vi "Main2.vi"() -> ()   [LabVIEW 2020]
uses:
  SuportVI2/Message Queue/Message Queue.lvlib
  SuportVI2/User Event - Stop/User Event - Stop.lvlib
  <vilib>/ErrorRing/Error Ring.xnode
  <vilib>/Utility/error.llb/Error Cluster From Error Code.vi
  <vilib>/userdefined/High Color/IMAQdx.ctl
  <vilib>/vision/Image Controls.llb/IMAQ Image.ctl
  <vilib>/vision/driver/NI_Vision_Acquisition_Software.lvlib
  Add/DAQ AO Sinus Config.ctl
  <vilib>/DAQmx/write.llb/DAQmx Write (Analog Wfm 1Chan NSamp).vi
  Desktop/QMH/ContAcqQMH_Lab/controls/Daqtypedef.ctl
  <vilib>/DAQmx/read.llb/DAQmx Read (Analog Wfm 1Chan NSamp).vi
panel:
  out "Waveform Graph":waveform(dbl)(graph)
  out "DB Data":T1
  out "Status Line 2":string
  in  "Generator Configuration":T2
  out "Image":T3(plugin-control)
  in  "Camera Config":cluster{"Camera Select":T4}
  in  "Exit":bool
  in  "Stop Camera":bool
  in  "Start Camera":bool
  out "Status Line":string
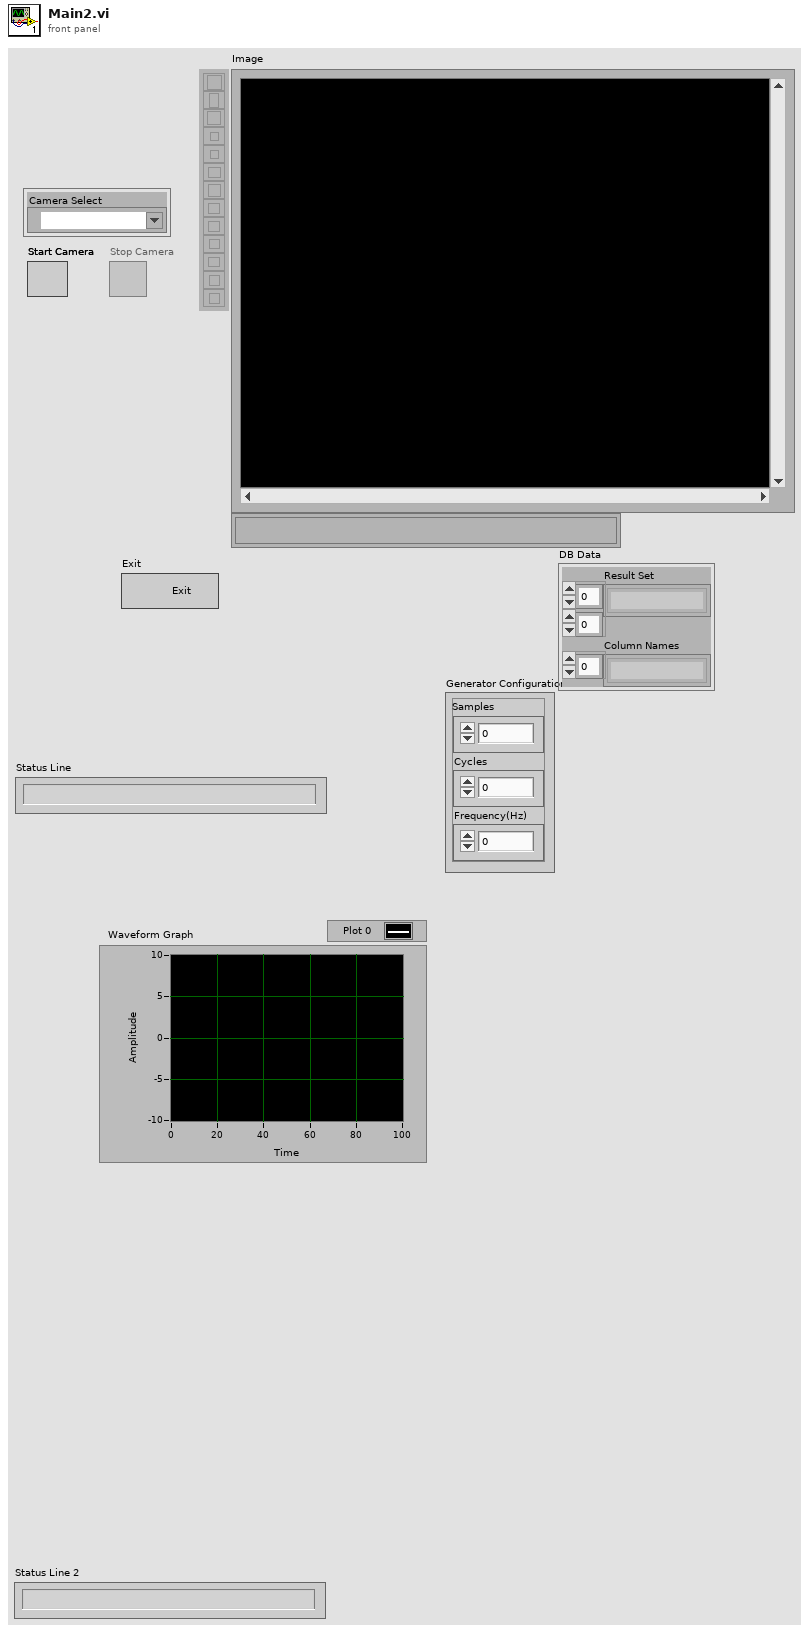
[diagram p1: front panel]
types:
  T1 = cluster{"Result Set":string[][], "Column Names":string[]}
  T2 = typedef "DAQ AO Sinus Config.ctl" = cluster{"Samples":i32, "Cycles":i32, "Frequency(Hz)":dbl}
  T3 = typedef "IMAQ Image.ctl" = refnum<image>
  T4 = typedef "IMAQdx.ctl" = refnum<k21>
  T5 = cluster{"DAQmx Channel":T2, "DAQmx Task":refnum<k21>, "DB Data":cluster{"Result Set":string[][], "Column Names":string[]}}
  T6 = typedef "Daqtypedef.ctl" = cluster{"PhysicalChanName":tag, "AI.Max":dbl, "AI.Min":dbl, "SampQuant.SampPerChan":i32, "SampClk.Rate":dbl}
  T7 = cluster{string, "configuration file path out":path, "Sin Samples":i32, "ID":i32, "Amplitude":dbl, "Frequency Cutoff":dbl, "Broadband Samples":i32, "Sin Samples rate":i32, "Sin AI Samples":i32, "DAQmxChannel":T6}
  T8 = cluster{"Image":cluster{"Image original":T3, "Image copy":T3, "Image Out":T3}, "Session Config":cluster{"Session":T4}, "Data":string}
  T9 = cluster{"Start Camera":refnum<vi>, "Stop Camera":refnum<vi>, "Exit":refnum<vi>, "Camera Conf":refnum<vi>, "Status Line":refnum<vi>, "Status Line Text":string, "Camera Select":refnum<vi>}
  T10 = cluster{"UI":refnum<queue>, "Camera":refnum<queue>, "Acquire":refnum<queue>, "SinusGen":refnum<queue>}
  T11 = cluster{"SampClk.Rate":dbl, "SampQuant.SampPerChan":i32, "AI.Min":dbl, "AI.Max":dbl, "PhysicalChanName":tag}
  T12 = typedef "Image Type" = u32
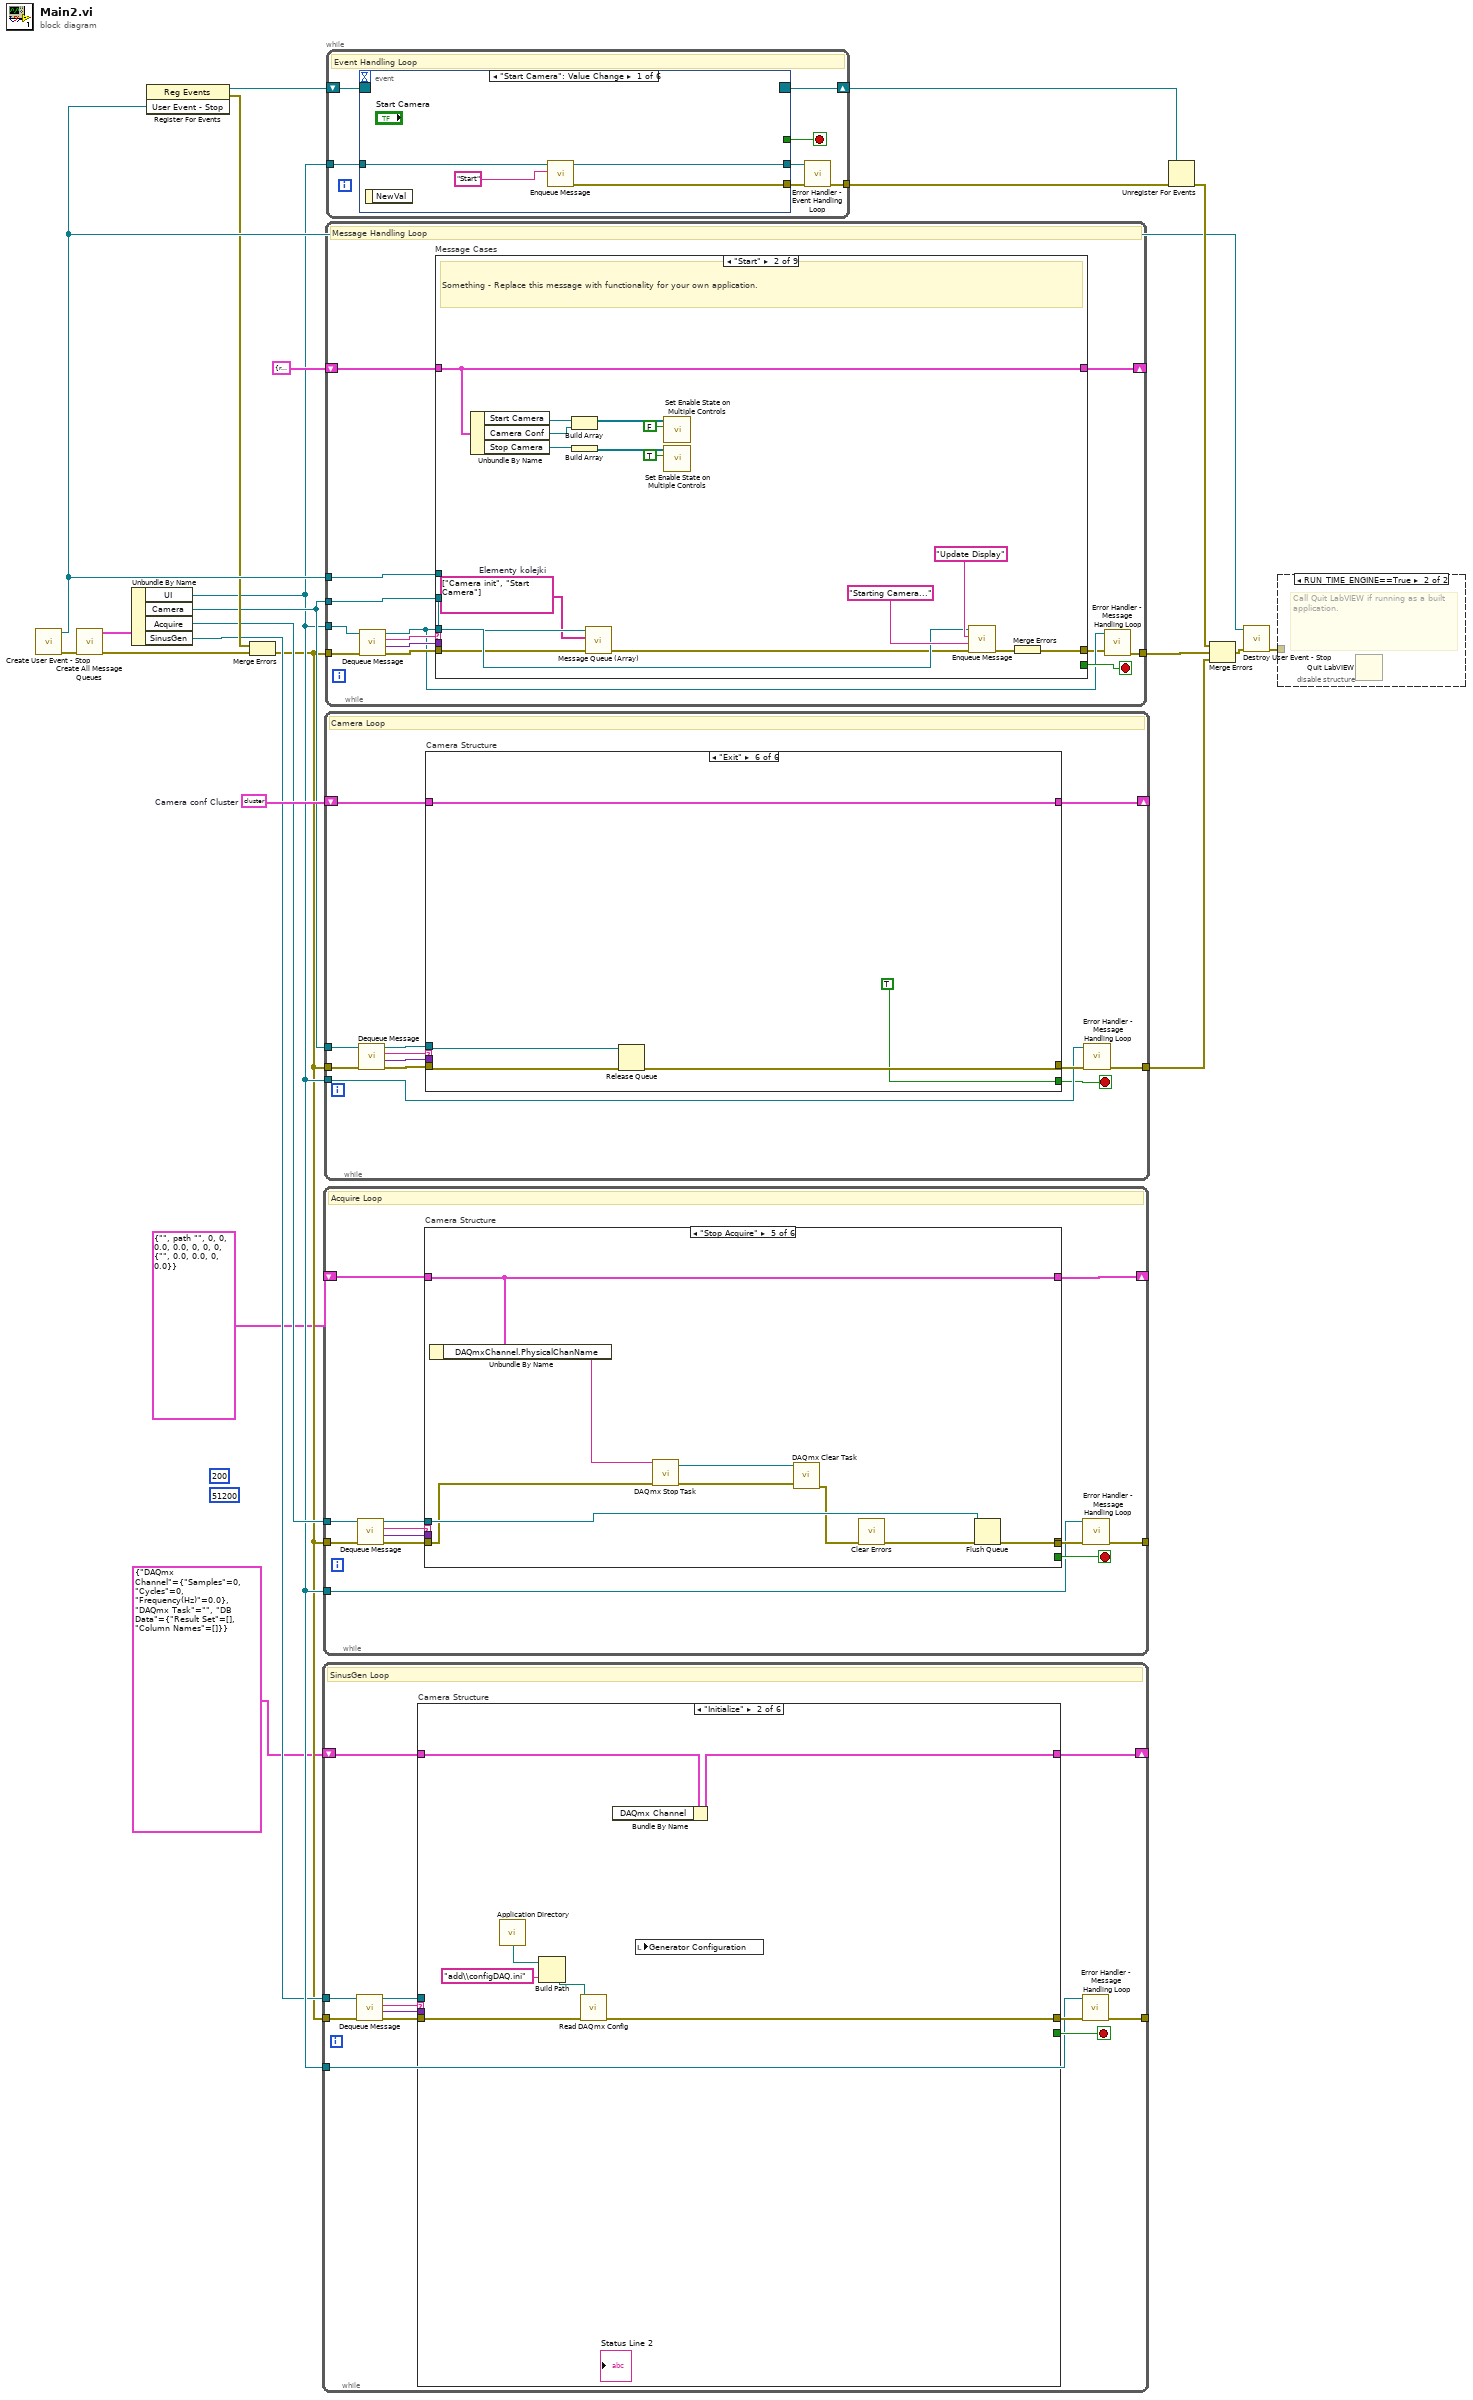
[diagram p0: block diagram]
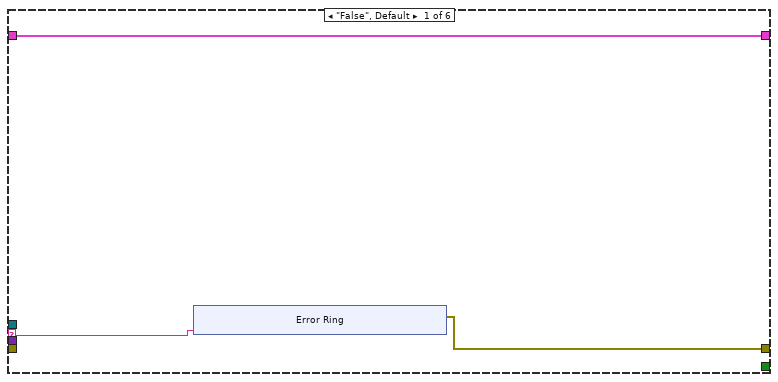
[diagram p2: hidden frame]
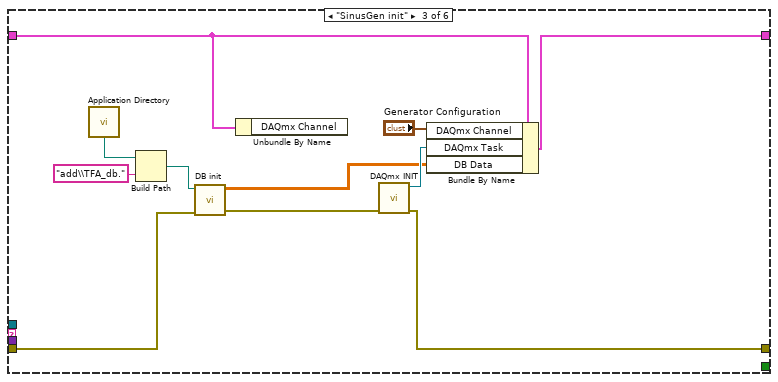
[diagram p3: hidden frame]
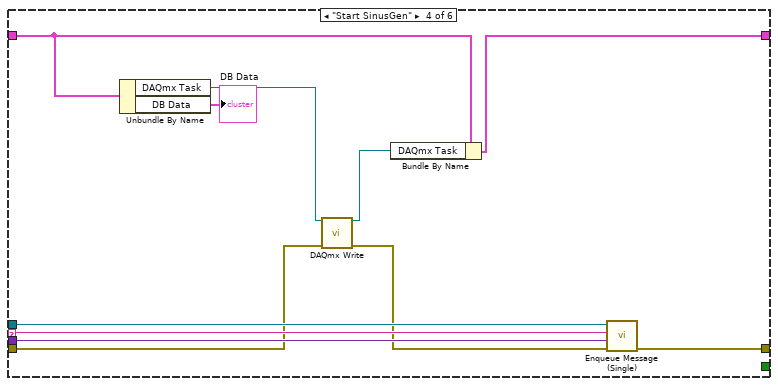
[diagram p4: hidden frame]
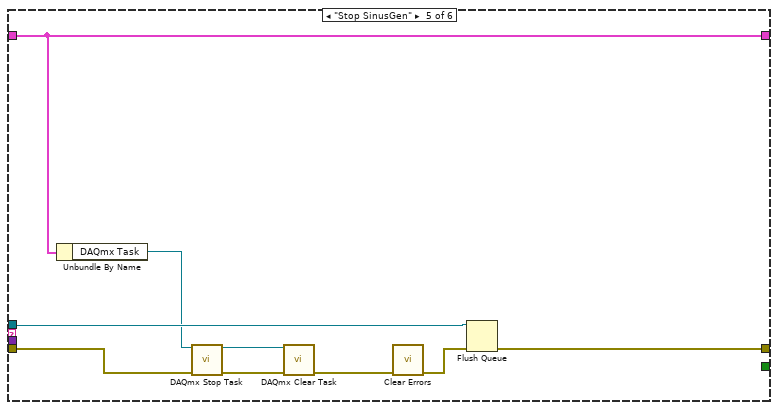
[diagram p5: hidden frame]
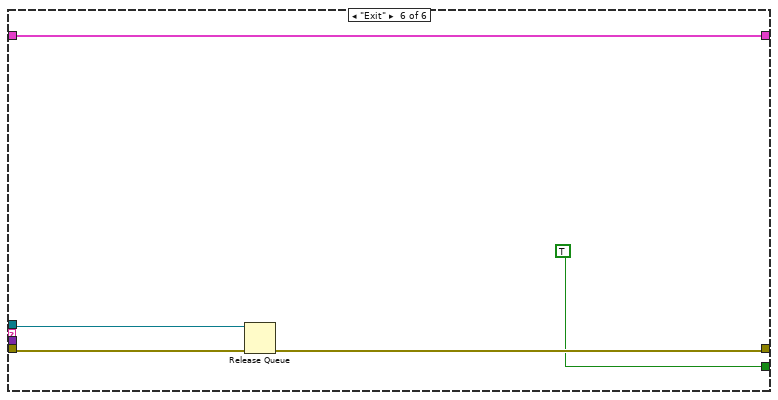
[diagram p6: hidden frame]
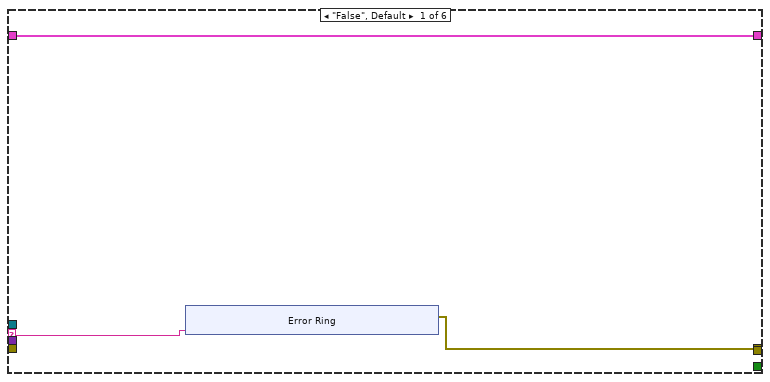
[diagram p7: hidden frame]
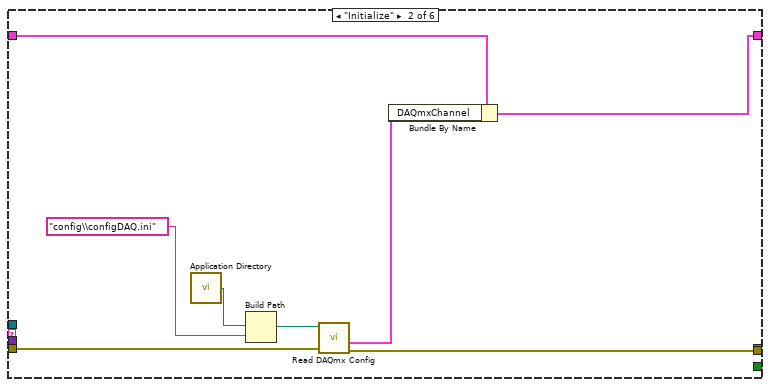
[diagram p8: hidden frame]
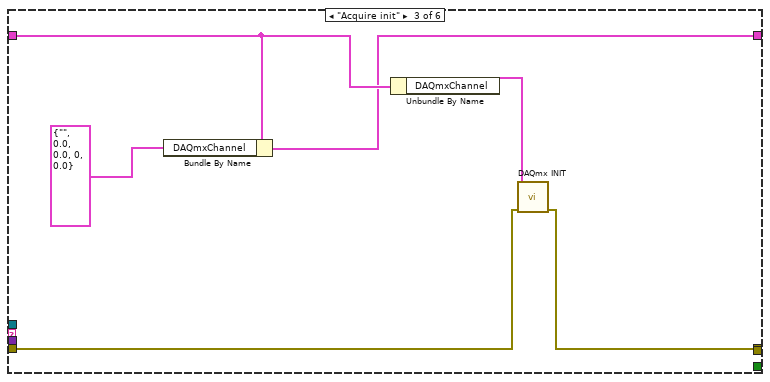
[diagram p9: hidden frame]
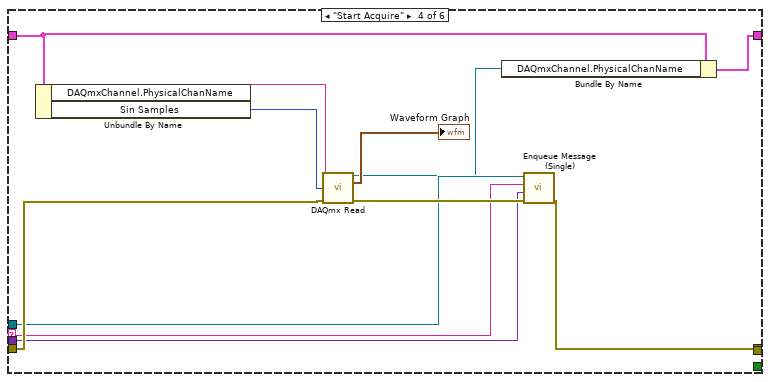
[diagram p10: hidden frame]
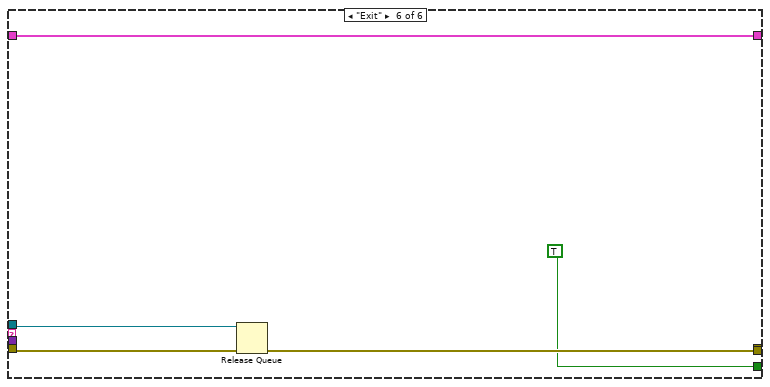
[diagram p11: hidden frame]
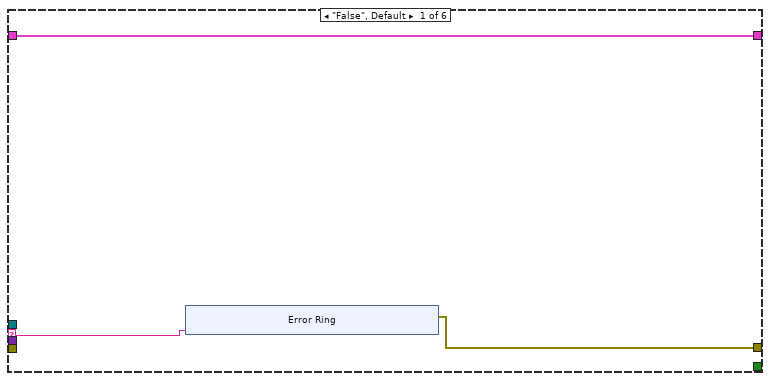
[diagram p12: hidden frame]
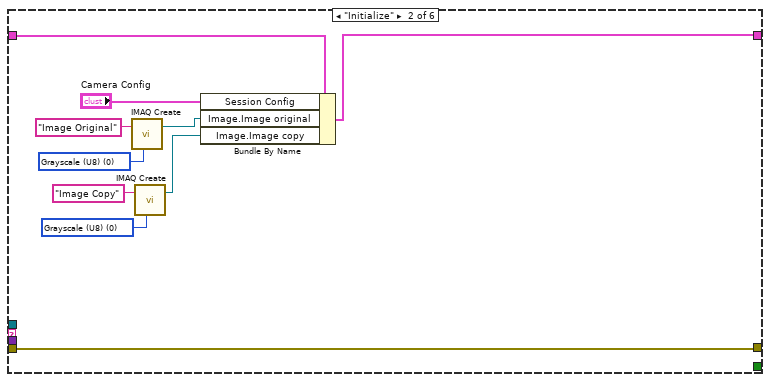
[diagram p13: hidden frame]
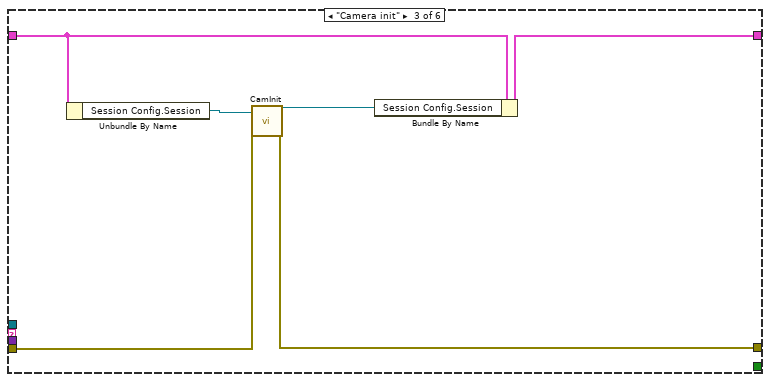
[diagram p14: hidden frame]
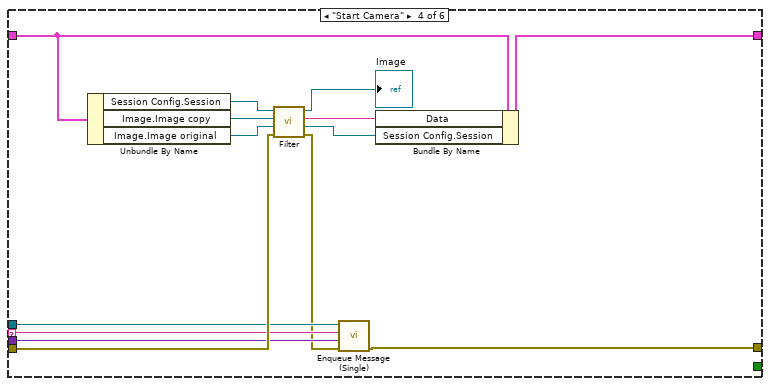
[diagram p15: hidden frame]
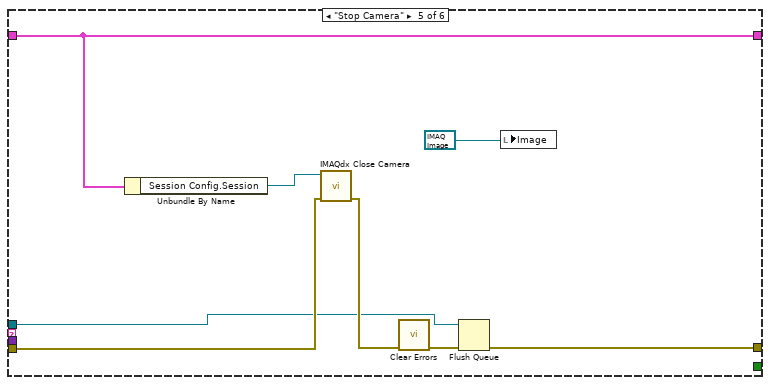
[diagram p16: hidden frame]
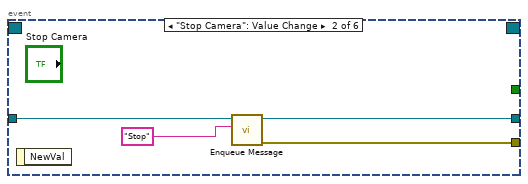
[diagram p18: hidden frame]
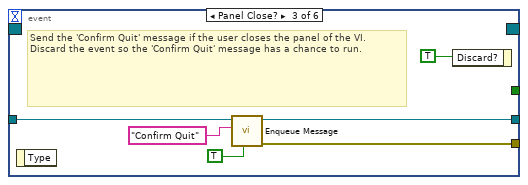
[diagram p19: hidden frame]
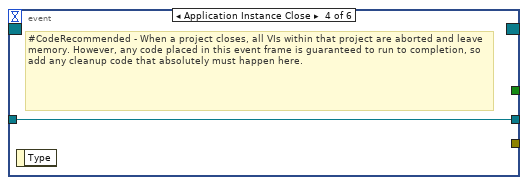
[diagram p20: hidden frame]
diagram:
  (unwired) 51200 ("Broadband Sample Rate")
  (unwired) 200 ("Broadband Delay")
  w9 = T8 {"Image"={"Image original"=refnum, "Image copy"=refnum, "Image Out"=refnum}, "Session Config"={"Session"=""}, "Data"=""}  # Camera conf Cluster
  n1 = call "Create User Event - Stop.vi"() -> ("error out"=w20:errorcluster, "User Event - Stop"=w13:refnum<user-event>)  [unwired: 10 in]
  n2 = call "Create All Message Queues.vi"("error in (no error)"=w20) -> ("error out"=w22:errorcluster, "Message Queues out"=w8:T10)  [unwired: 9 in]
  n3 = Unbundle By Name(w8) -> ("UI"=w5:refnum<queue>, "Camera"=w7:refnum<queue>, "Acquire"=w6:refnum<queue>, "SinusGen"=w4:refnum<queue>)
  n4 = register-events(w13) -> (reference out=w14:refnum<event-registration>, error out=w12:errorcluster)  [unwired: 2 in]
  n5 = Merge Errors(w12, w22) -> (w3:errorcluster)
  n6 = while {
    shift-right: [w24] -> _
    shift-left: T5 {"DAQmx Channel"={"Samples"=0, "Cycles"=0, "Frequency(Hz)"=0.0}, "DAQmx Task"="", "DB Data"={"Result Set"=[], "Column Names"=[]}} -> [w23]
    tunnel: [w34] -> _
    tunnel: w4 -> [w31]
    tunnel: w3 -> [w26]
    tunnel: w5 -> [w25]
    stop <- w28 stop-if-true
    # "SinusGen Loop"
    n7 = call "Dequeue Message.vi"("error in (no error)"=w26, "Message Queue"=w31) -> ("error out"=w33:errorcluster, "Message Data"=w29:variant, "Message"=w27:string, "dup Message Queue"=w30:refnum<queue>)  [unwired: 6 in]
    n8 = case "Camera Structure" shown="\"Initialize\"" w27 {
      selector: w27 -> [w36 _ _ w72 _ _]
      tunnel: [w37 w47 w62 w70 w81 w86] -> w32
      tunnel: w33 -> [_ w48 w57 w69 w75 w85]
      tunnel: w30 -> [_ _ _ w73 w80 w87]
      tunnel: w29 -> [_ _ _ w71 _ _]
      tunnel: [_ _ _ _ _ TRUE] -> w28
      tunnel: [w35 w45 w60 w64 w77 w83] -> w24
      tunnel: w23 -> [w35 w46 w61 w65 w77 w83]
      frame "False", Default {
        n9 = xnode "Error Ring"("parameter 0"=w36) -> ("error out"=w37:errorcluster)
      }
      frame "Initialize" {
        n10 = call <vilib>:"Application Directory.vi"() -> ("Application Directory"=w51:path)
        n11 = Build Path(base path=w51, name or relative path="add\\configDAQ.ini") -> (appended path=w49:path)
        n12 = call "Read DAQmx Config.vi"("error in (no error)"=w48, "configuration file path"=w49) -> ("error out"=w47:errorcluster)  [unwired: 7 in, 2 out]
        n13 = Bundle By Name(cluster=w46) -> (w45:T5)  [unwired: 1 in]
        n14 = local read "Generator Configuration"() -> ()  [unwired: 1 in]
      }
      frame "SinusGen init" {
        n15 = call <vilib>:"Application Directory.vi"() -> ("Application Directory"=w54:path)
        n16 = Build Path(base path=w54, name or relative path="add\\TFA_db.") -> (appended path=w52:path)
        n17 = call "DB init.vi"("error in (no error)"=w57, "DB path"=w52) -> ("error out"=w56:errorcluster, "DB Data"=w55:dbl[][])  [unwired: 8 in]
        n18 = Unbundle By Name(w61) -> ()  [unwired: 1 out]
        n19 = call "DAQmx INIT.vi"("error in"=w56) -> ("error out"=w62:errorcluster, "task out"=w59:refnum<k21>)  [unwired: 9 in]
        n20 = Bundle By Name(cluster=w61, "DAQmx Channel"="Generator Configuration", "DAQmx Task"=w59, "DB Data"=w55) -> (w60:T5)
      }
      frame "Start SinusGen" {
        n21 = Unbundle By Name(w65) -> ("DAQmx Task"=w67:refnum<k21>, "DB Data"=→"DB Data":T1)
        n22 = call-poly <vilib>:"DAQmx Write.vi"("task/channels in"=w67, "error in"=w69) -> ("task out"=w66:refnum<k21>, "error out"=w68:errorcluster)  [unwired: 11 in, 1 out]
        n23 = Bundle By Name(cluster=w65, "DAQmx Task"=w66) -> (w64:T5)
        n24 = call "Enqueue Message (Single).vi"("error in (no error)"=w68, "Message Data"=w71, "Message"=w72, "Message Queue"=w73) -> ("error out"=w70:errorcluster)  [unwired: 6 in, 1 out]
      }
      frame "Stop SinusGen" {
        n25 = Unbundle By Name(w77) -> ("DAQmx Task"=w76:refnum<k21>)
        n26 = call <vilib>:"DAQmx Stop Task.vi"("task/channels in"=w76, "error in"=w75) -> ("task out"=w79:refnum<k21>, "error out"=w78:errorcluster)  [unwired: 12 in]
        n27 = call <vilib>:"DAQmx Clear Task.vi"("task in"=w79, "error in"=w78) -> ("error out"=w74:errorcluster)  [unwired: 13 in]
        n28 = call <vilib>:"Clear Errors.vi"("error in (no error)"=w74) -> ("error out"=w82:errorcluster)  [unwired: 5 in, 1 out]
        n29 = Flush Queue(queue=w80, error in (no error)=w82) -> (error out=w81:errorcluster)  [unwired: 2 out]
      }
      frame "Exit" {
        n30 = Release Queue(queue=w87, error in (no error)=w85) -> (error out=w86:errorcluster)  [unwired: 1 in, 2 out]
      }
    }
    n31 = call "Error Handler - Message Handling Loop.vi"("error in (no error)"=w32, "Message Queue"=w25) -> ("dup error in"=w34:errorcluster)  [unwired: 8 in, 1 out]
  }
  n32 = while {
    shift-right: [w89] -> _
    shift-left: T7 {"", "configuration file path out"=path "", "Sin Samples"=0, "ID"=0, "Amplitude"=0.0, "Frequency Cutoff"=0.0, "Broadband Samples"=0, "Sin Samples rate"=0, "Sin AI Samples"=0, "DAQmxChannel"={"PhysicalChanName"="", "AI.Max"=0.0, "AI.Min"=0.0, "SampQuant.SampPerChan"=0, "SampClk.Rate"=0.0}} -> [w88]
    tunnel: [w99] -> _
    tunnel: w6 -> [w96]
    tunnel: w3 -> [w91]
    tunnel: w5 -> [w90]
    stop <- w93 stop-if-true
    # "Acquire Loop"
    n33 = call "Dequeue Message.vi"("error in (no error)"=w91, "Message Queue"=w96) -> ("error out"=w98:errorcluster, "Message Data"=w94:variant, "Message"=w92:string, "dup Message Queue"=w95:refnum<queue>)  [unwired: 6 in]
    n34 = case "Camera Structure" shown="\"Stop Acquire\"" w92 {
      selector: w92 -> [w101 _ _ w127 _ _]
      tunnel: [w102 _ w122 w135 w143 w148] -> w97
      tunnel: w98 -> [_ w115 w123 w132 w137 w147]
      tunnel: w95 -> [_ _ _ w129 w142 w149]
      tunnel: w94 -> [_ _ _ w128 _ _]
      tunnel: [_ _ _ _ _ TRUE] -> w93
      tunnel: [w100 w112 w119 w134 w141 w145] -> w89
      tunnel: w88 -> [w100 w113 w120 w133 w141 w145]
      tunnel: [_ w114 _ _ _ _] -> _
      frame "False", Default {
        n35 = xnode "Error Ring"("parameter 0"=w101) -> ("error out"=w102:errorcluster)
      }
      frame "Initialize" {
        n36 = call <vilib>:"Application Directory.vi"() -> ("Application Directory"=w117:path)
        n37 = Build Path(base path=w117, name or relative path="config\\configDAQ.ini") -> (appended path=w116:path)
        n38 = call "Read DAQmx Config.vi"("error in (no error)"=w115, "configuration file path"=w116) -> ("error out"=w114:errorcluster, "data"=w110:T11)  [unwired: 7 in, 1 out]
        n39 = Bundle By Name(cluster=w113, "DAQmxChannel"=w110) -> (w112:T7)
      }
      frame "Acquire init" {
        n40 = Bundle By Name(cluster=w120, "DAQmxChannel"=T6 {"PhysicalChanName"="", "AI.Max"=0.0, "AI.Min"=0.0, "SampQuant.SampPerChan"=0, "SampClk.Rate"=0.0}) -> (w119:T7)
        n41 = Unbundle By Name(w120) -> ("DAQmxChannel"=w121:T6)
        n42 = call "DAQmx INIT.vi"("error in"=w123, "DAQmxChannel"=w121) -> ("error out"=w122:errorcluster)  [unwired: 8 in, 1 out]
      }
      frame "Start Acquire" {
        n43 = Unbundle By Name(w133) -> ("DAQmxChannel.PhysicalChanName"=w125:tag, "Sin Samples"=w130:i32)
        n44 = call-poly <vilib>:"DAQmx Read.vi"("task/channels in"=w125, "number of samples per channel"=w130, "error in"=w132) -> ("task out"=w124:refnum<k21>, "data"=→"Waveform Graph":waveform(dbl), "error out"=w131:errorcluster)  [unwired: 10 in]
        n45 = Bundle By Name(cluster=w133, "DAQmxChannel.PhysicalChanName"=w124) -> (w134:T7)
        n46 = call "Enqueue Message (Single).vi"("error in (no error)"=w131, "Message Data"=w128, "Message"=w127, "Message Queue"=w129) -> ("error out"=w135:errorcluster)  [unwired: 6 in, 1 out]
      }
      frame "Stop Acquire" {
        n47 = Unbundle By Name(w141) -> ("DAQmxChannel.PhysicalChanName"=w136:tag)
        n48 = call <vilib>:"DAQmx Stop Task.vi"("task/channels in"=w136, "error in"=w137) -> ("task out"=w139:refnum<k21>, "error out"=w138:errorcluster)  [unwired: 12 in]
        n49 = call <vilib>:"DAQmx Clear Task.vi"("task in"=w139, "error in"=w138) -> ("error out"=w140:errorcluster)  [unwired: 13 in]
        n50 = call <vilib>:"Clear Errors.vi"("error in (no error)"=w140) -> ("error out"=w144:errorcluster)  [unwired: 5 in, 1 out]
        n51 = Flush Queue(queue=w142, error in (no error)=w144) -> (error out=w143:errorcluster)  [unwired: 2 out]
      }
      frame "Exit" {
        n52 = Release Queue(queue=w149, error in (no error)=w147) -> (error out=w148:errorcluster)  [unwired: 1 in, 2 out]
      }
    }
    n53 = call "Error Handler - Message Handling Loop.vi"("error in (no error)"=w97, "Message Queue"=w90) -> ("dup error in"=w99:errorcluster)  [unwired: 8 in, 1 out]
  }
  n54 = while {
    shift-right: [w153] -> _
    shift-left: w9 -> [w156]
    tunnel: [w161] -> w10
    tunnel: w3 -> [w160]
    tunnel: w5 -> [w157]
    tunnel: w7 -> [w155]
    stop <- w151 stop-if-true
    # "Camera Loop"
    n55 = call "Dequeue Message.vi"("error in (no error)"=w160, "Message Queue"=w155) -> ("error out"=w159:errorcluster, "Message Data"=w152:variant, "Message"=w150:string, "dup Message Queue"=w154:refnum<queue>)  [unwired: 6 in]
    n56 = case "Camera Structure" shown="\"Exit\"" w150 {
      selector: w150 -> [w162 _ _ w192 _ _]
      tunnel: [w164 w181 w184 w189 w204 w212] -> w158
      tunnel: w159 -> [_ w181 w185 w201 w209 w211]
      tunnel: w156 -> [w163 w179 w183 w197 w208 w214]
      tunnel: w154 -> [_ _ _ w193 w203 w213]
      tunnel: [w163 w178 w182 w194 w208 w214] -> w153
      tunnel: w152 -> [_ _ _ w191 _ _]
      tunnel: [_ _ _ _ _ TRUE] -> w151
      frame "False", Default {
        n57 = xnode "Error Ring"("parameter 0"=w162) -> ("error out"=w164:errorcluster)
      }
      frame "Initialize" {
        w173 = T12 0 items=["Grayscale (U8)", "Grayscale (I16)", "Grayscale (SGL)", "Complex (CSG)", "RGB (U32)", "HSL (U32)", "RGB (U64)", "Grayscale (U16)"] ("Image Type")
        w176 = T12 0 items=["Grayscale (U8)", "Grayscale (I16)", "Grayscale (SGL)", "Complex (CSG)", "RGB (U32)", "HSL (U32)", "RGB (U64)", "Grayscale (U16)"] ("Image Type")
        n58 = call "IMAQ Create"("Image Name"="Image Original", "Image Type"=w173) -> ("New Image"=w172:T3)  [unwired: 3 in, 1 out]
        n59 = call "IMAQ Create"("Image Name"="Image Copy", "Image Type"=w176) -> ("New Image"=w175:T3)  [unwired: 3 in, 1 out]
        n60 = Bundle By Name(cluster=w179, "Session Config"="Camera Config", "Image.Image original"=w172, "Image.Image copy"=w175) -> (w178:T8)
      }
      frame "Camera init" {
        n61 = Unbundle By Name(w183) -> ("Session Config.Session"=w187:T4)
        n62 = call "CamInit.vi"("error in (no error)"=w185, "Refnum in"=w187) -> ("error out"=w184:errorcluster, "Refnum out"=w186:T4)  [unwired: 8 in]
        n63 = Bundle By Name(cluster=w183, "Session Config.Session"=w186) -> (w182:T8)
      }
      frame "Start Camera" {
        n64 = Unbundle By Name(w197) -> ("Session Config.Session"=w200:T4, "Image.Image copy"=w199:T3, "Image.Image original"=w198:T3)
        n65 = call "Filter.vi"("error in"=w201, "Image original"=w198, "Image copy"=w199, "Session Config"=w200) -> ("error out"=w190:errorcluster, "Session Out"=w195:T4, "Data"=w196:string, "Image Out"=→"Image":T3)  [unwired: 4 in]
        n66 = call "Enqueue Message (Single).vi"("error in (no error)"=w190, "Message Data"=w191, "Message"=w192, "Message Queue"=w193) -> ("error out"=w189:errorcluster)  [unwired: 6 in, 1 out]
        n67 = Bundle By Name(cluster=w197, "Data"=w196, "Session Config.Session"=w195) -> (w194:T8)
      }
      frame "Stop Camera" {
        n68 = Unbundle By Name(w208) -> ("Session Config.Session"=w207:T4)
        n69 = call <vilib>:"IMAQdx Close Camera.vi"("error in"=w209, "Session In"=w207) -> ("error out"=w205:errorcluster)  [unwired: 9 in]
        n70 = call <vilib>:"Clear Errors.vi"("error in (no error)"=w205) -> ("error out"=w206:errorcluster)  [unwired: 5 in, 1 out]
        n71 = Flush Queue(queue=w203, error in (no error)=w206) -> (error out=w204:errorcluster)  [unwired: 2 out]
        n72 = local write "Image"(T3 refnum ("Image")) -> ()
      }
      frame "Exit" {
        n73 = Release Queue(queue=w213, error in (no error)=w211) -> (error out=w212:errorcluster)  [unwired: 1 in, 2 out]
      }
    }
    n74 = call "Error Handler - Message Handling Loop.vi"("error in (no error)"=w158, "Message Queue"=w157) -> ("dup error in"=w161:errorcluster)  [unwired: 8 in, 1 out]
  }
  n75 = while {
    tunnel: w5 -> [w219]
    shift-right: [w226] -> _
    shift-left: T9 {"Start Camera"=refnum, "Stop Camera"=refnum, "Exit"=refnum, "Camera Conf"=refnum, "Status Line"=refnum, "Status Line Text"="", "Camera Select"=refnum} -> [w227]
    tunnel: w13 -> [w224]
    tunnel: w3 -> [w223]
    tunnel: [w217] -> w21
    tunnel: w7 -> [w215]
    stop <- w225 stop-if-true
    # "Message Handling Loop"
    n76 = call "Dequeue Message.vi"("error in (no error)"=w223, "Message Queue"=w219) -> ("error out"=w222:errorcluster, "Message Data"=w220:variant, "Message"=w221:string, "dup Message Queue"=w218:refnum<queue>)  [unwired: 6 in]
    n77 = case "Message Cases" shown="\"Start\"" w221 {
      selector: w221 -> [_ _ _ _ _ _ _ _ w318]
      tunnel: w218 -> [w233 w254 w274 _ _ w293 _ w317 _]
      tunnel: w222 -> [w240 w251 w271 w281 w290 w297 w300 w308 _]
      tunnel: [w241 w258 w276 w282 w284 w295 w298 w314 w319] -> w216
      tunnel: w227 -> [w239 w249 w259 w283 w289 w296 w299 w306 w320]
      tunnel: [w238 w249 w259 w283 w289 w296 w299 w306 w320] -> w226
      tunnel: [_ _ _ _ _ _ _ TRUE _] -> w225
      tunnel: w220 -> [_ _ _ w280 w288 _ _ _ _]
      tunnel: w224 -> [_ _ _ _ _ _ _ w313 _]
      tunnel: w215 -> [_ w253 w269 _ _ _ _ w311 _]
      frame "Initialize" {
        w232 = "Initialization Completed" ("Initial Message")
        # "Initialize - All initialization work should take place in this message, since other loops can potentially enqueue messages that execute immediately after this one."
        n78 = control-ref of="Start Camera"() -> (w237:refnum<vi>)
        n79 = control-ref of="Stop Camera"() -> (w228:refnum<vi>)
        n80 = control-ref of="Exit"() -> (w235:refnum<vi>)
        n81 = control-ref of="Camera Config"() -> (w231:refnum<vi>)
        n82 = control-ref of="Status Line"() -> (w236:refnum<vi>)
        n83 = Build Array(w228) -> (w229:refnum<vi>[])
        n84 = Bundle By Name(cluster=w239, "Start Camera"=w237, "Stop Camera"=w228, "Status Line"=w236, "Exit"=w235, "Status Line Text"=w232, "Camera Select"=w231) -> (w238:T9)
        n85 = call "Set Enable State on Multiple Controls.vi"("Enable?"=FALSE, "Controls"=w229) -> ()  [unwired: 10 in]
        n86 = call-poly "Enqueue Message.vi"("error in (no error)"=w240, "Message Data"=w232, "Message"="Update Display", "Message Queue"=w233) -> ("error out"=w241:errorcluster)  [unwired: 6 in, 1 out]
      }
      frame "Start" {
        w252 = string[] ["Camera init", "Start Camera"]  # Elementy kolejki
        # "Something - Replace this message with functionality for your own application."
        n87 = Unbundle By Name(w249) -> ("Start Camera"=w243:refnum<vi>, "Camera Conf"=w244:refnum<vi>, "Stop Camera"=w245:refnum<vi>)
        n88 = Build Array(w243, w244) -> (w248:refnum<vi>[])
        n89 = Build Array(w245) -> (w247:refnum<vi>[])
        n90 = call "Message Queue (Array).vi"("error in (no error)"=w251, "Message Array"=w252, "Message Queue"=w253) -> ("error out"=w250:errorcluster)  [unwired: 7 in, 1 out]
        n91 = call "Set Enable State on Multiple Controls.vi"("Enable?"=FALSE, "Controls"=w248) -> ()  [unwired: 10 in]
        n92 = call "Set Enable State on Multiple Controls.vi"("Enable?"=TRUE, "Controls"=w247) -> ()  [unwired: 10 in]
        n93 = call-poly "Enqueue Message.vi"("error in (no error)"=w250, "Message Data"="Starting Camera..." ("\"Do Something\" button pressed"), "Message"="Update Display", "Message Queue"=w254) -> ("error out"=w257:errorcluster)  [unwired: 6 in, 1 out]
        n94 = Merge Errors(w257) -> (w258:errorcluster)
      }
      frame "Stop" {
        # "Something Else - Replace this message with functionality for your own application."
        n95 = Unbundle By Name(w259) -> ("Start Camera"=w261:refnum<vi>, "Camera Conf"=w262:refnum<vi>, "Stop Camera"=w263:refnum<vi>)
        n96 = Build Array(w261, w262) -> (w266:refnum<vi>[])
        n97 = Build Array(w263) -> (w265:refnum<vi>[])
        n98 = call "Set Enable State on Multiple Controls.vi"("Enable?"=TRUE, "Controls"=w266) -> ()  [unwired: 10 in]
        n99 = call "Set Enable State on Multiple Controls.vi"("Enable?"=FALSE, "Controls"=w265) -> ()  [unwired: 10 in]
        n100 = call-poly "Enqueue Message.vi"("Priority Message? (F)"=TRUE, "error in (no error)"=w271, "Message"="Stop Camera", "Message Queue"=w269) -> ("error out"=w270:errorcluster)  [unwired: 6 in, 1 out]
        n101 = call-poly "Enqueue Message.vi"("error in (no error)"=w270, "Message Data"="Camera Stopped" ("\"Do Something Else\" button pressed"), "Message"="Update Display", "Message Queue"=w274) -> ("error out"=w275:errorcluster)  [unwired: 6 in, 1 out]
        n102 = Merge Errors(w275) -> (w276:errorcluster)
      }
      frame "Update Display" {
        # "#CodeRecommended - If you wish to decouple the Message Handling Loop from your user interface, consider creating User Events (like the \"Stop\" event in this VI) to message the Event Handling Loop whenever the user interface needs updating."
        # "Update Display - Convert the message data to a string to display in the Data Display indicator."
        n103 = Variant To Data(error in=w281, type="", Variant=w280) -> (data=→"Status Line":string, error out=w278:errorcluster)
        n104 = Merge Errors(w278) -> (w282:errorcluster)
      }
      frame "Error" {
        # "#CodeRecommended - If you ever change the name of this \"Error\" message, you'll need to update the name in the Check Loop Error.vi as well."
        # "#CodeRecommended - Consider creating a system for logging errors in some way. These errors are for notification purposes only. Handling of specific errors should be performed in the message frames that generated the error."
        # "Error - Display an error dialog. This message is sent by the \"Error Handler\" VIs at the end of other loops in this application."
        n105 = Variant To Data(error in=w290, type=errorcluster {"status"=FALSE, "code"=0, "source"=""} ("error constant"), Variant=w288) -> (data=w286:errorcluster, error out=w285:errorcluster)
        n106 = call <vilib>:"Simple Error Handler.vi"("error in (no error)"=w286) -> ()  [unwired: 4 in, 5 out]
        n107 = Merge Errors(w285) -> (w284:errorcluster)
      }
      frame "Confirm Quit" {
        # "#CodeNeeded - If you want to provide an \"Are you sure\" dialog (or some other notification) before the application exits, place that code here. This message is typically sent from a Panel Close? event."
        # "Confirm Quit - Message that can confirm whether or not the user wants to exit the application."
        n108 = call-poly "Enqueue Message.vi"("Priority Message? (F)"=TRUE, "error in (no error)"=w297, "Message"="Exit", "Message Queue"=w293) -> ("error out"=w294:errorcluster)  [unwired: 6 in, 1 out]
        n109 = Merge Errors(w294) -> (w295:errorcluster)
      }
      frame "---Copy This Frame---" {
        # "Duplicate this frame when creating new messages.  Change this comment in the duplicated frame to describe this message."
        n110 = Merge Errors(w300) -> (w298:errorcluster)
      }
      frame "Exit" {
        # "Stop the VI"
        # "Exit - Exit the application."
        n111 = call "Enqueue Message (Single).vi"("Priority Message? (F)"=TRUE, "error in (no error)"=w308, "Message"="Exit", "Message Queue"=w311) -> ("error out"=w307:errorcluster)  [unwired: 6 in, 1 out]
        n112 = Unbundle By Name(w306) -> ("Start Camera"=w303:refnum<vi>, "Stop Camera"=w302:refnum<vi>, "Camera Conf"=w301:refnum<vi>)
        n113 = call "Fire User Event - Stop.vi"("User Event - Stop"=w313) -> ("error out"=w312:errorcluster)  [unwired: 10 in]
        n114 = Release Queue(queue=w317, error in (no error)=w307) -> (error out=w315:errorcluster)  [unwired: 1 in, 2 out]
        n115 = Build Array(w303, w302, w301) -> (w304:refnum<vi>[])
        n116 = Merge Errors(w312, w315) -> (w314:errorcluster)
        n117 = call "Set Enable State on Multiple Controls.vi"("Enable?"=TRUE, "Controls"=w304) -> ()  [unwired: 10 in]
      }
      frame Default {
        # "'Default' case only runs if there is a message that isn't defined in any of the other cases.  Output a programming error."
        n118 = xnode "Error Ring"("parameter 0"=w318) -> ("error out"=w319:errorcluster)
      }
    }
    n119 = call "Error Handler - Message Handling Loop.vi"("error in (no error)"=w216, "Message Queue"=w218) -> ("dup error in"=w217:errorcluster)  [unwired: 8 in, 1 out]
  }
  n120 = while {
    tunnel: w5 -> [w334]
    shift-right: [w332] -> w17
    shift-left: w14 -> [w333]
    tunnel: [w328] -> w15
    stop <- w330 stop-if-true
    # "Event Handling Loop"
    n121 = event shown="[0] \"Start Camera\": Value Change" {
      selector: w333 -> [_ _ _ _ _ _]
      dyn-events: [_ _ _ _ _ _] -> w332
      timeout: _ -> [_ _ _ _ _ _]
      tunnel: [_ _ _ _ _ TRUE ("Discard?")] -> w330
      tunnel: w334 -> [w338 w342 w347 w349 w354 w357]
      tunnel: [w335 w339 w346 _ w353 _] -> w331
      tunnel: [w337 w341 w345 w349 w352 w357] -> w329
      event "Start Camera": Value Change {
        n122 = event-data() -> ()  [unwired: 1 in, 1 out]
        n123 = call-poly "Enqueue Message.vi"("Message"="Start", "Message Queue"=w338) -> ("error out"=w335:errorcluster, "dup Message Queue"=w337:refnum<queue>)  [unwired: 8 in]
      }
      event "Stop Camera": Value Change {
        n124 = event-data() -> ()  [unwired: 1 in, 1 out]
        n125 = call-poly "Enqueue Message.vi"("Message"="Stop", "Message Queue"=w342) -> ("error out"=w339:errorcluster, "dup Message Queue"=w341:refnum<queue>)  [unwired: 8 in]
      }
      event Panel Close? {
        # "Send the 'Confirm Quit' message if the user closes the panel of the VI. Discard the event so the 'Confirm Quit' message has a chance to run."
        n126 = event-data() -> ()  [unwired: 1 in, 1 out]
        n127 = call-poly "Enqueue Message.vi"("Priority Message? (F)"=TRUE, "Message"="Confirm Quit", "Message Queue"=w347) -> ("error out"=w346:errorcluster, "dup Message Queue"=w345:refnum<queue>)  [unwired: 7 in]
        n128 = event-data("Discard?"=TRUE) -> ()  [unwired: 1 in, 1 out]
      }
      event Application Instance Close {
        # "#CodeRecommended - When a project closes, all VIs within that project are aborted and leave memory. However, any code placed in this event frame is guaranteed to run to completion, so add any cleanup code that absolutely must happen here."
        n129 = event-data() -> ()  [unwired: 1 in, 1 out]
      }
      event "Exit": Value Change {
        n130 = event-data() -> ()  [unwired: 1 in, 1 out]
        n131 = call-poly "Enqueue Message.vi"("Priority Message? (F)"=TRUE, "Message"="Exit", "Message Queue"=w354) -> ("error out"=w353:errorcluster, "dup Message Queue"=w352:refnum<queue>)  [unwired: 7 in]
      }
      event User Event {
        # "The Message Handling Loop processed an \"Exit\" message, which fired this event to stop the Event Handling Loop."
        n132 = event-data() -> ()  [unwired: 1 in, 1 out]
        n133 = local write "Status Line"("Exiting application" ("VI Stopped")) -> ()
      }
    }
    n134 = call "Error Handler - Event Handling Loop.vi"("error in (no error)"=w331, "Message Queue"=w329) -> ("dup error in"=w328:errorcluster)  [unwired: 8 in, 1 out]
  }
  n135 = Unregister For Events(event registration refnum=w17, error in=w15) -> (error out=w18:errorcluster)
  n136 = Merge Errors(w18, w21, w10) -> (w19:errorcluster)
  n137 = call "Destroy User Event - Stop.vi"("error in (no error)"=w19, "User Event - Stop"=w13) -> ("error out"=w16:errorcluster)  [unwired: 9 in]
  n138 = disable-structure shown="RUN_TIME_ENGINE==True" {
    disable-tunnel: w16 -> [_ _]
    frame condition #0 (active) {
    }
    frame condition #1 {
      # "Call Quit LabVIEW if running as a built application."
      n139 = Quit LabVIEW() -> ()  [unwired: 1 in]
    }
  }
